vi "Square Wave Generator (FPGA).vi"() -> ()   [LabVIEW 2012]
doc: "This VI uses the Square Wave Generator VI to create signals for the outputs. The frequency, phase offset, duty cycle, offset, and amplitude of the signals can be programmatically changed from the host VI."
uses:
  <vilib>/rvi/eio/common/nirviEmuTemplateMethod_errors.vi
  <vilib>/eio/EIONode/EIONode.xnode
panel:
  in  "Square wave":T1={"frequency (periods/tick)"=0.9999999997671694, "phase offset (periods)"=0.0, "amplitude"=32767, "offset"=0, "duty cycle (periods)"=0.9999999997671694}
  in  "reset":bool
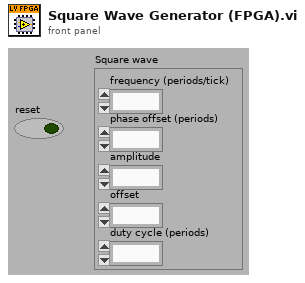
[diagram p1: front panel]
types:
  T1 = cluster{"frequency (periods/tick)":fxp<+,32,0>, "phase offset (periods)":fxp<+,32,0>, "amplitude":i16, "offset":i16, "duty cycle (periods)":fxp<+,32,0>}
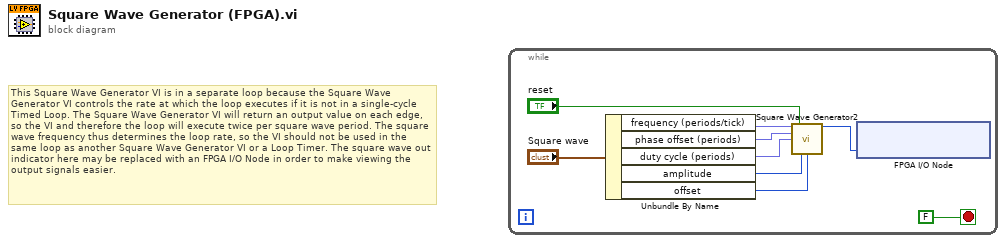
[diagram p0: block diagram]
diagram:
  # "This Square Wave Generator VI is in a separate loop because the Square Wave Generator VI controls the rate at which the loop executes if it is not in a single-cycle Timed Loop. The Square Wave Generator VI will return an output value on each edge, so the VI and therefore the loop will execute twice per square wave period. The square wave frequency thus determines the loop rate, so the VI should not be used in the same loop as another Square Wave Generator VI or a Loop Timer. The square wave out indicator here may be replaced with an FPGA I/O Node in order to make viewing the output signals easier."
  n1 = while {
    stop <- FALSE stop-if-true
    n2 = Unbundle By Name("Square wave") -> ("frequency (periods/tick)"=w5:fxp<+,32,0>, "phase offset (periods)"=w4:fxp<+,32,0>, "duty cycle (periods)"=w3:fxp<+,32,0>, "amplitude"=w8:i16, "offset"=w9:i16)
    n3 = call "Square Wave Generator2"("frequency (periods/tick)"=w5, "reset"="reset", "phase offset (periods)"=w4, "duty cycle (periods)"=w3, "amplitude"=w8, "offset"=w9) -> ("square wave out"=w1:i16)  [unwired: 9 in]
    n4 = xnode "FPGA I/O Node"("Connector0/AO7"=w1) -> ()  [unwired: 1 in, 1 out]
  }
